vi "SA5G_measureEVM.vi"(8 "error in":errorcluster, 11 "VISA in":refnum<visa-resource-name>) -> (0 "error out":errorcluster, 2 "SA_Resp":string, 3 "VISA out":refnum<visa-resource-name>)   [LabVIEW 2020, in "Keysight.lvlib"]
uses:
  Keysight.lvlib
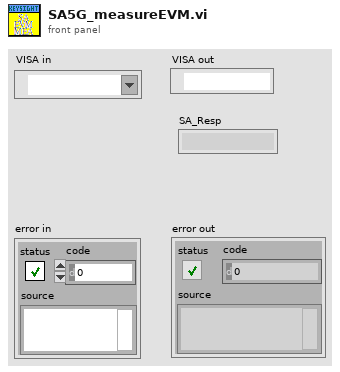
[diagram p1: front panel]
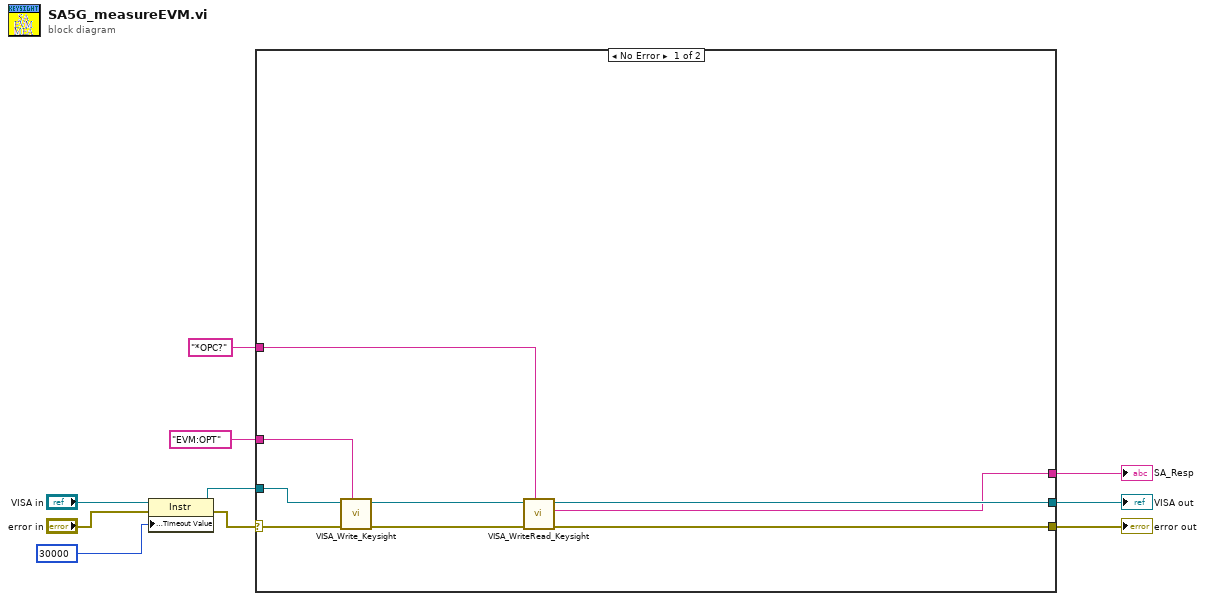
[diagram p0: block diagram]
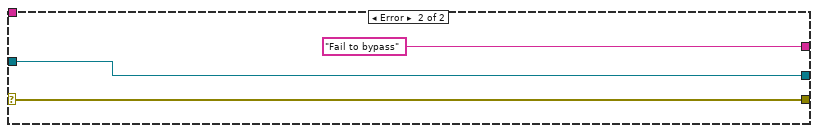
[diagram p2: hidden frame]
diagram:
  n1 = property on="Property Node" class="Instr"(reference="VISA in", error in="error in", "General Settings:Timeout Value"=u32 30000) -> (reference out=w2:refnum<visa-resource-name>, error out=w3:errorcluster)
  n2 = case shown="No Error" w3 {
    selector: w3 -> [w15 w22]
    tunnel: [w19 w22] -> w8
    tunnel: [w18 w20] -> w9
    tunnel: [w17 "Fail to bypass" ("Response")] -> w10
    tunnel: "*OPC?" ("write buffer") -> [w16 _]
    tunnel: w2 -> [w13 w20]
    tunnel: "EVM:OPT" ("write buffer") -> [w11 _]
    frame No Error {
      n3 = call "VISA_Write_Keysight.vi"("VISA CMD"=w11, "error in"=w15, "VISA in"=w13) -> ("error out"=w12:errorcluster, "VISA out"=w14:refnum<visa-resource-name>)  [unwired: 7 in]
      n4 = call "VISA_WriteRead_Keysight.vi"("VISA_CMD"=w16, "error in"=w12, "VISA in"=w14) -> ("error out"=w19:errorcluster, "Response"=w17:string, "VISA out"=w18:refnum<visa-resource-name>)  [unwired: 6 in]
    }
    frame Error {
    }
  }
  "SA_Resp" <- w10
  "VISA out" <- w9
  "error out" <- w8
